vi "BINARY READ AND WRITE.vi"() -> ()   [LabVIEW 2018]
panel:
  out "data":cluster{"A":bool, "B":dbl, "C":bool}
  in  "Cluster":cluster{"A":bool, "B":dbl, "C":bool}
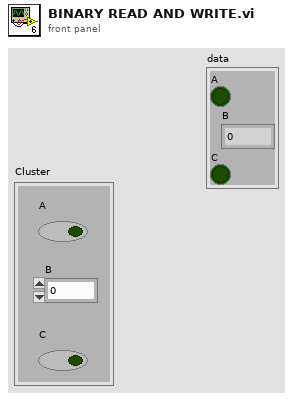
[diagram p1: front panel]
types:
  T1 = enum16{"open", "replace", "create", "open or create", "replace or create", "replace or create with confirmation"}
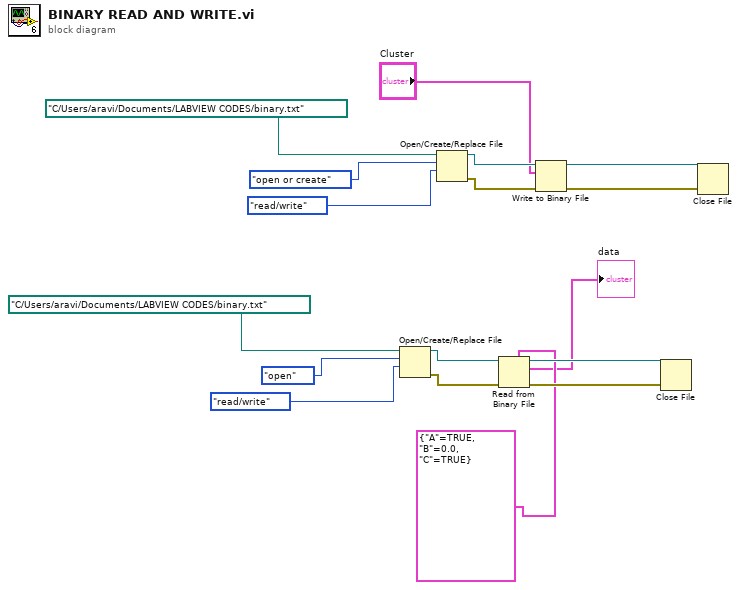
[diagram p0: block diagram]
diagram:
  n1 = Open/Create/Replace File(file path (use dialog)=path "C:/Users/aravi/Documents/LABVIEW CODES/binary.txt", operation (0:open)=T1."open", access (0:read/write)=enum16{"read/write", "read-only", "write-only"}."read/write") -> (refnum out=w6:refnum<file>, error out=w5:errorcluster)  [unwired: 3 in, 1 out]
  n2 = Open/Create/Replace File(file path (use dialog)=path "C:/Users/aravi/Documents/LABVIEW CODES/binary.txt", operation (0:open)=T1."open or create", access (0:read/write)=enum16{"read/write", "read-only", "write-only"}."read/write") -> (refnum out=w14:refnum<file>, error out=w13:errorcluster)  [unwired: 3 in, 1 out]
  n3 = Read from Binary File(5:cluster{"A":bool, "B":dbl, "C":bool} {"A"=TRUE, "B"=0.0, "C"=TRUE}, 8:w5, 11:w6) -> (0:w4:errorcluster, 2:→"data":cluster{"A":bool, "B":dbl, "C":bool}, 3:w3:refnum<file>)  [unwired: 3 in, 1 out]
  n4 = Write to Binary File(file (use dialog)=w14, data="Cluster", error in=w13) -> (refnum out=w11:refnum<file>, error out=w12:errorcluster)  [unwired: 3 in, 1 out]
  n5 = Close File(refnum=w3, error in=w4) -> ()  [unwired: 2 out]
  n6 = Close File(refnum=w11, error in=w12) -> ()  [unwired: 2 out]
